vi "Framework Test.vi"() -> ()   [LabVIEW 2017]
uses:
  Builds/Data Sharing Framework/Current/Data Sharing Framework Core/DSF Core.lvlibp/Configuration/Public/Controls/DSF Direction.ctl
  Builds/Data Sharing Framework/Current/Data Sharing Framework Core/DSF Core.lvlibp/Configuration/Public/Controls/DSF Timing Info.ctl
  Builds/Data Sharing Framework/Current/Data Sharing Framework Core/DSF Core.lvlibp/Configuration/Public/Controls/DSF Settings Info.ctl
  Builds/Data Sharing Framework/Current/Data Sharing Framework Core/DSF Core.lvlibp/Configuration/Public/Controls/DSF Data Type.ctl
  <vilib>/Platform/TimedLoop/XDataNode/timing_clust.ctl
  <vilib>/Platform/TimedLoop/XDataNode/nitl_modes.ctl
  <vilib>/Platform/TimedLoop/XDataNode/wakeup.ctl
  Builds/Data Sharing Framework/Current/Data Sharing Framework Core/DSF Core.lvlibp/Engine/Classes/Debug/FIFO Flags/FIFO Flags.lvclass
  Builds/Data Sharing Framework/Current/Data Sharing Framework Core/DSF Core.lvlibp/Engine/Classes/Debug/Debug Flags/Debug Flags.lvclass
  Builds/Data Sharing Framework/Current/Data Sharing Framework Core/DSF Core.lvlibp/Engine/Classes/Framework/Framework.lvclass
  <vilib>/NI/Memory Manager/Classes/Pointer/Pointer.lvclass/Pointer.ctl
  <vilib>/NI/Memory Manager/Classes/Pointer/Public/New/New (4B).vi
  <vilib>/NI/Memory Manager/Classes/Pointer/Public/Write/Write (0D U32).vi
  <vilib>/NI/Memory Manager/Classes/Pointer/Public/New/New (1B).vi
  <vilib>/NI/Memory Manager/Classes/Pointer/Public/Write/Write (0D Bool).vi
  <vilib>/NI/Memory Manager/Classes/Pointer/Public/New/New (8B).vi
  <vilib>/NI/Memory Manager/Classes/Pointer/Public/Read/Read (0D I32).vi
  <vilib>/NI/Memory Manager/Classes/Pointer/Public/Read/Read (0D U32).vi
  <vilib>/NI/Memory Manager/Classes/Pointer/Public/Read/Read (0D Bool).vi
  <vilib>/NI/Memory Manager/Classes/Pointer/Public/Write/Write (0D I32).vi
  <vilib>/NI/Memory Manager/Classes/Pointer/Private/Allocate.vi
  <vilib>/NI/Memory Manager/Classes/Pointer/Public/Write (No Check)/Write (No Check 0D U32).vi
  <vilib>/NI/Memory Manager/Classes/Pointer/Protected/Parameter Checking/Check Null Pointer.vi
  <vilib>/NI/Memory Manager/Classes/Pointer/Protected/Parameter Checking/Check Subset.vi
  <vilib>/NI/Memory Manager/Classes/Pointer/Public/Write (No Check)/Write (No Check 0D Bool).vi
  <vilib>/NI/Memory Manager/Classes/Pointer/Public/Read (No Check)/Read (No Check 0D I32).vi
  <vilib>/NI/Memory Manager/Classes/Pointer/Public/Read (No Check)/Read (No Check 0D U32).vi
  <vilib>/NI/Memory Manager/Classes/Pointer/Public/Read (No Check)/Read (No Check 0D Bool).vi
  <vilib>/NI/Memory Manager/Classes/Pointer/Public/Write (No Check)/Write (No Check 0D I32).vi
  <vilib>/NI/Memory Manager/Classes/Pointer/API/Accessors/Set Address.vi
  <vilib>/NI/Memory Manager/Classes/Pointer/API/Accessors/Set Size.vi
  <vilib>/NI/Memory Manager/Classes/Pointer/Private/Set Internal.vi
  <vilib>/NI/Memory Manager/Classes/Pointer/Protected/Errors.vi
  <vilib>/NI/Memory Manager/Classes/Pointer/Protected/Error VIs/Null Pointer.vi
  <vilib>/NI/Memory Manager/Classes/Pointer/Protected/Error VIs/Out of Bounds.vi
  <vilib>/NI/Memory Manager/Classes/Pointer/Protected/Error Building/Create Error.vi
  <vilib>/NI/Memory Manager/VIs/Write String into Source.vi
  <vilib>/NI/Memory Manager/Classes/Pointer/Protected/Error Building/Write Pointer Size.vi
  <vilib>/NI/Memory Manager/VIs/Write Number into Source.vi
  <vilib>/NI/Memory Manager/VIs/VIs for Poly/Write U64 into Source.vi
  <vilib>/NI/Memory Manager/Constants/Constants.vi
  <vilib>/NI/Memory Manager/Constants/Library Name.vi
  <vilib>/NI/Memory Manager/Classes/Pointer/Protected/Error Building/Get Error Info.vi
  <vilib>/NI/Memory Manager/VIs/Create Error Cluster.vi
  <vilib>/NI/Memory Manager/VIs/VIs for Poly/Create Error Cluster (256B).vi
  <vilib>/NI/Memory Manager/VIs/Set Error Status.vi
  <vilib>/NI/Memory Manager/VIs/Set Error Code.vi
  <vilib>/NI/Memory Manager/VIs/Set Error Source.vi
  <vilib>/NI/Memory Manager/Classes/Pointer/Pointer.lvclass
  <vilib>/platform/TimedLoop/XDataNode/XDataNode.xnode
  <vilib>/Platform/TimedLoop/XDataNode/XDNodeRunTimeDep.lvlib
  Builds/Data Sharing Framework/Current/Data Sharing Framework Core/DSF Core.lvlibp/Engine/Classes/Status/Framework Status.lvclass
  Builds/Data Sharing Framework/Current/Data Sharing Framework Core/DSF Core.lvlibp/Engine/Classes/Status/Framework Performance.lvclass
  Builds/Data Sharing Framework/Current/Data Sharing Framework Core/DSF Core.lvlibp/Configuration/Configuration Session.lvclass
  Builds/Data Sharing Framework/Current/Data Sharing Framework Core/DSF Core.lvlibp
panel:
  in  "Components Path":path=path "C:/Builds/Data Sharing Framework/Windows/32/Transceivers"
  in  "UDP Rx max size":i32=800
  in  "UDP Rx ports":u16[](array[numeric])=[60000, 60001, 60002, 60003]
  in  "Plugins":T5(array[cluster])=[{"plugin class"="UDP", "group configs"=[{"direction"=enum."Tx", "timing"={"priority"=100, "decimation"=1, "offset"=0}, "settings"=[], "transfer configs"=[{"random types?"=FALSE, "non-random type"=enum."DBL", "channel count"=100, "settings"=[{"key"="Destination Address", "value"="localhost"}, {"key"="Destination Port", "value"="60000"}]}]}, {"direction"=enum."Tx", "timing"={"priority"=100, "decimation"=2, "offset"=0}, "settings"=[], "transfer configs"=[{"random types?"=FALSE, "non-random type"=enum."DBL", "channel count"=100, "settings"=[{"key"="Destination Address", "value"="localhost"}, {"key"="Destination Port", "value"="60001"}]}]}, {"direction"=enum."Tx", "timing"={"priority"=100, "decimation"=3, "offset"=0}, "settings"=[], "transfer configs"=[{"random types?"=FALSE, "non-random type"=enum."DBL", "channel count"=100, "settings"=[{"key"="Destination Address", "value"="localhost"}, {"key"="Destination Port", "value"="60002"}]}]}, {"direction"=enum."Tx", "timing"={"priority"=100, "decimation"=4, "offset"=0}, "settings"=[], "transfer configs"=[{"random types?"=FALSE, "non-random type"=enum."DBL", "channel count"=100, "settings"=[{"key"="Destination Address", "value"="localhost"}, {"key"="Destination Port", "value"="60003"}]}]}], "plugin timing"={"priority"=100, "decimation"=1, "offset"=0}, "settings"=[{"key"="Local Port", "value"="50000"}], "thread count"=1}]
  in  "Infinite Timeouts":bool=TRUE
  out "Framework Error":errorcluster
  out "Tx duration":u32 format="%d us"
  out "Rx duration":u32 format="%d us"
  out "Actual Frequency":dbl format="%.0pHz"
  in  "Configuration Path":path=path "C:/github/data-sharing-framework/Testing/test.dsf"
  out "Framework Iteration":i32 format="%d cycles"
  out "Actual Period":u32 format="%d us"
  in  "Target PCL Period":u32=10000 caption="Target Period" format="%d us"
  in  "stop":bool
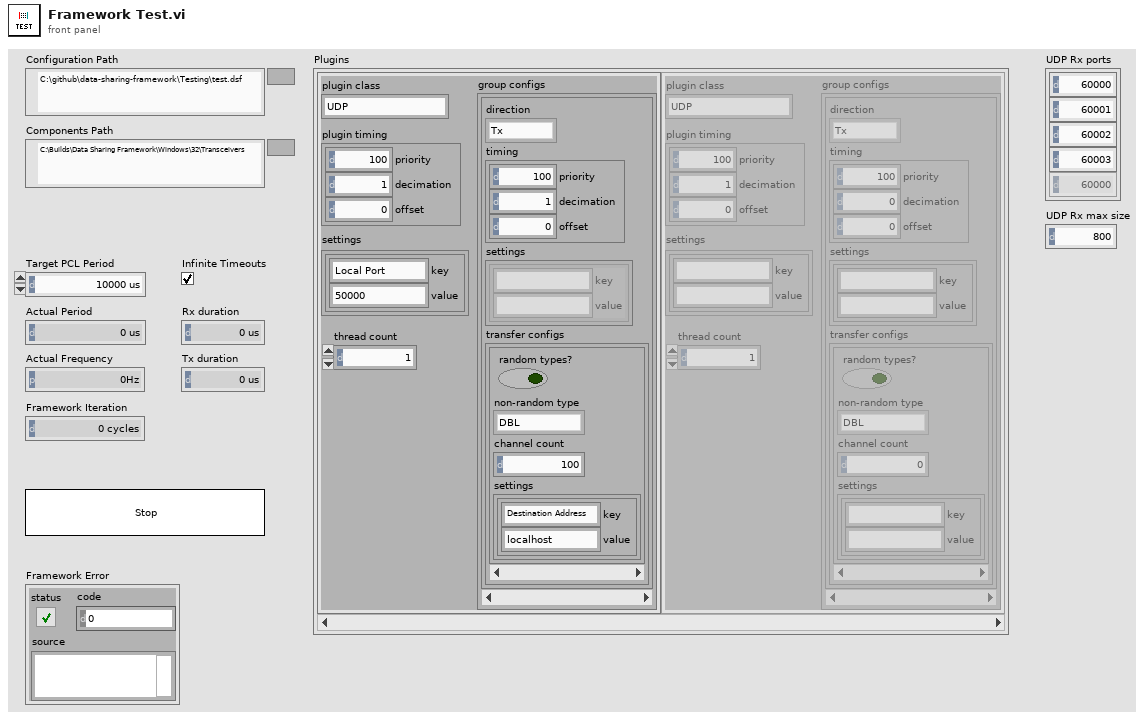
[diagram p1: front panel]
types:
  T1 = typedef "DSF Core.lvlibp/DSF Direction.ctl" = enum8{"Tx", "Rx"}
  T2 = typedef "DSF Core.lvlibp/DSF Timing Info.ctl" = cluster{"priority":u64, "decimation":u64, "offset":u64}
  T3 = typedef "DSF Core.lvlibp/DSF Settings Info.ctl" = cluster{"key":string, "value":string}[]
  T4 = typedef "DSF Core.lvlibp/DSF Data Type.ctl" = enum8{"Bool", "SGL", "DBL", "I8", "I16", "I32", "I64", "U8", "U16", "U32", "U64"}
  T5 = cluster{"plugin class":string, "group configs":cluster{"direction":T1, "timing":T2, "settings":T3, "transfer configs":cluster{"random types?":bool, "non-random type":T4, "channel count":i32, "settings":T3}[]}[], "plugin timing":T2, "settings":T3, "thread count":i32}[]
  T6 = typedef "DSF Core.lvlibp/DSF Engine Framework Configuration.ctl" = cluster{"Plugins":T7[]}
  T7 = typedef "DSF Core.lvlibp/DSF Engine Plugin Configuration.ctl" = cluster{"name":string, "class":string, "cycle timing":T2, "Transfer Groups":T8[], "settings":T3, "thread count":i32}
  T8 = typedef "DSF Core.lvlibp/DSF Engine Transfer Group Configuration.ctl" = cluster{"name":string, "direction":T1, "cycle timing":T2, "Transfers":T9[], "settings":T3}
  T9 = typedef "DSF Core.lvlibp/DSF Engine Transfer Configuration.ctl" = cluster{"name":string, "byte order":T10, "channel configurations":T11[], "settings":T3}
  T10 = typedef "DSF Core.lvlibp/DSF Byte Order.ctl" = enum8{"big-endian", "little-endian"}
  T11 = typedef "DSF Core.lvlibp/DSF Engine Channel Configuration.ctl" = cluster{"engine offset":u64, "name":string, "data type":T4, "count":u64, "buffer offset":u64}
  T12 = typedef "XDNodeRunTimeDep.lvlib/timing_clust.ctl" = cluster{"Expected End [f-1]":u64, "Actual End [f-1]":u64, "Finished Late? [f-1]":bool, "Expected End [i-1]":u64, "Actual End [i-1]":u64, "Finished Late? [i-1]":bool, "Expected Start [i]":u64, "Actual Start [i]":u64, "Expected Start [f]":u64, "Actual Start [f]":u64, "Source Name":string, "Structure Name":string, "Period":i64, "Deadline":i64, "Offset":i64, "Start":i64, "Priority":i32, "Timeout":i32, "Mode":T13, "Wakeup Reason":T14, "Error":errorcluster, "Source Type":string, "Secondary Source Type":string, "Global End Time":u64, "Global Start Time":u64, "Frame Duration":u64, "Iteration Duration":u64, "Assigned CPU":i32, "I/O Scan Engine Mode":u32}
  T13 = typedef "XDNodeRunTimeDep.lvlib/nitl_modes.ctl" = enum32{"No Change", "Process missed periods, maintain original phase", "Discard missed periods, maintain original phase", "Process missed periods, ignore original phase", "Discard missed periods, ignore original phase"}
  T14 = typedef "XDNodeRunTimeDep.lvlib/wakeup.ctl" = enum32{"Normal", "Aborted", "Asynchronous wakeup", "Timing source error", "Timed loop error", "Timeout"}
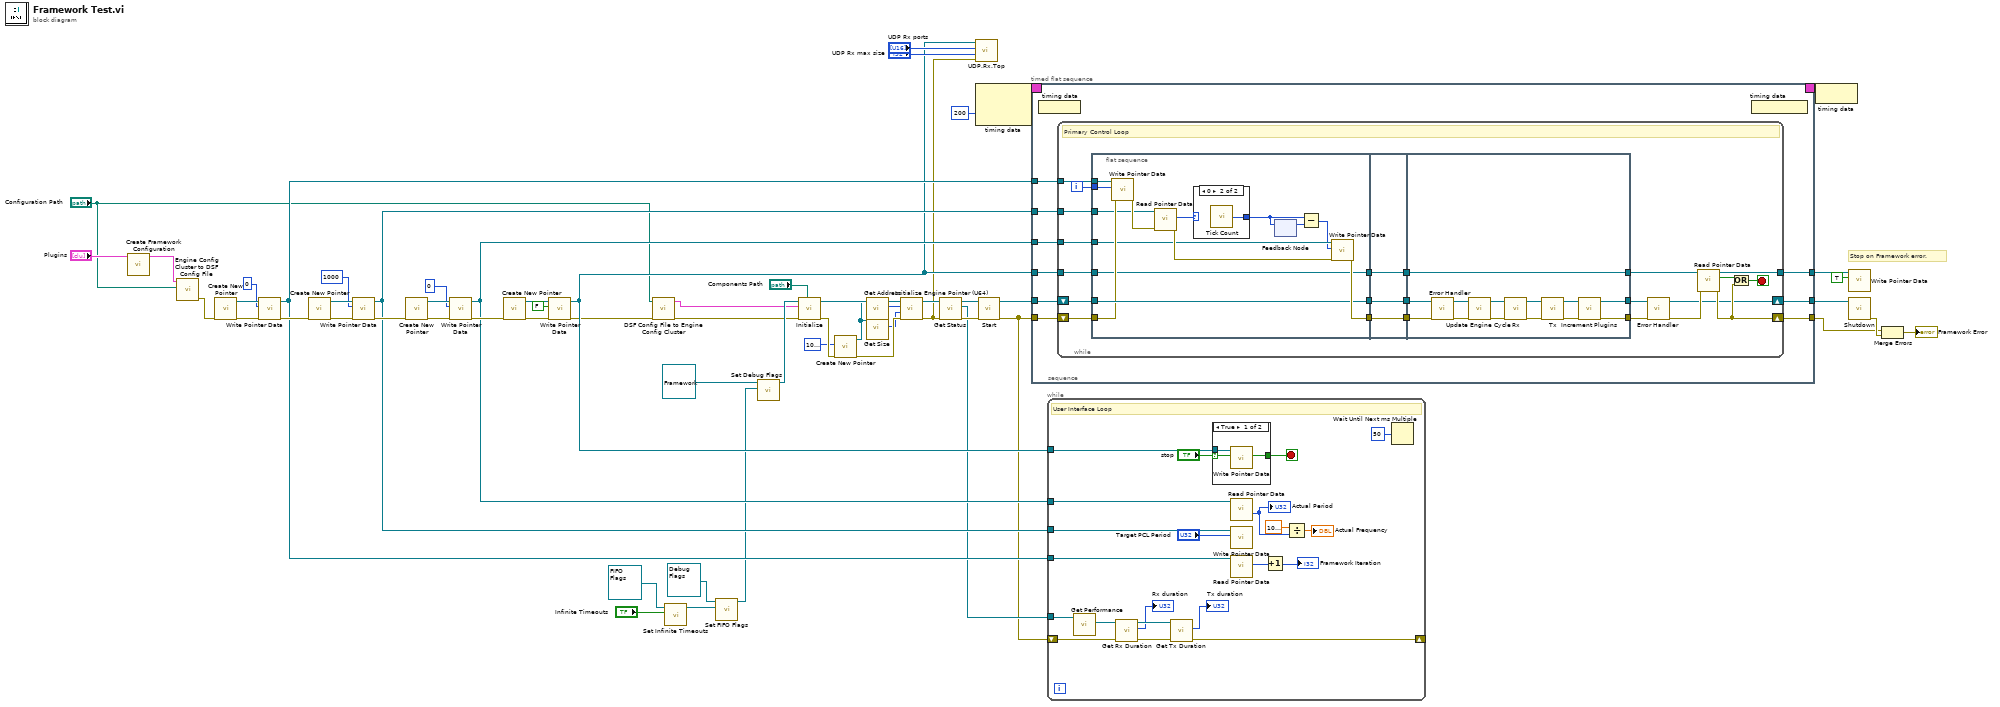
[diagram p0: block diagram]
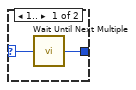
[diagram p2: hidden frame]
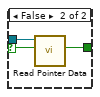
[diagram p3: hidden frame]
diagram:
  # "Stop on Framework error."
  n1 = call "Create Framework Configuration.vi"("Plugins"="Plugins") -> ("Framework Configuration"=w12:T6)  [unwired: 10 in]
  n2 = call "Engine Config Cluster to DSF Config File.vi"("dsf configuration file path"="Configuration Path", "framework configuration"=w12) -> ("error out"=w10:errorcluster)  [unwired: 9 in]
  n3 = call-poly <vilib>:"Create New Pointer.vi"("error in (no error)"=w10) -> ("error out"=w44:errorcluster, "Pointer"=w45:refnum<class "Pointer.lvclass">)  [unwired: 9 in]
  n4 = call-poly <vilib>:"Write Pointer Data.vi"("error in (no error)"=w44, "value"=u32 0, "Pointer in"=w45) -> ("error out"=w43:errorcluster, "Pointer out"=w42:refnum<class "Pointer.lvclass">)  [unwired: 5 in, 2 out]
  n5 = call-poly <vilib>:"Create New Pointer.vi"("error in (no error)"=w43) -> ("error out"=w51:errorcluster, "Pointer"=w52:refnum<class "Pointer.lvclass">)  [unwired: 9 in]
  n6 = call-poly <vilib>:"Write Pointer Data.vi"("error in (no error)"=w51, "value"=u32 1000, "Pointer in"=w52) -> ("error out"=w50:errorcluster, "Pointer out"=w46:refnum<class "Pointer.lvclass">)  [unwired: 5 in, 2 out]
  n7 = call-poly <vilib>:"Create New Pointer.vi"("error in (no error)"=w50) -> ("error out"=w49:errorcluster, "Pointer"=w53:refnum<class "Pointer.lvclass">)  [unwired: 9 in]
  n8 = call-poly <vilib>:"Write Pointer Data.vi"("error in (no error)"=w49, "value"=u32 0, "Pointer in"=w53) -> ("error out"=w48:errorcluster, "Pointer out"=w47:refnum<class "Pointer.lvclass">)  [unwired: 5 in, 2 out]
  n9 = call-poly <vilib>:"Create New Pointer.vi"("error in (no error)"=w48) -> ("error out"=w56:errorcluster, "Pointer"=w55:refnum<class "Pointer.lvclass">)  [unwired: 9 in]
  n10 = call-poly <vilib>:"Write Pointer Data.vi"("error in (no error)"=w56, "value"=FALSE, "Pointer in"=w55) -> ("error out"=w9:errorcluster, "Pointer out"=w37:refnum<class "Pointer.lvclass">)  [unwired: 5 in, 2 out]
  n11 = call "DSF Config File to Engine Config Cluster.vi"("error in (no error)"=w9, "dsf configuration file path"="Configuration Path") -> ("error out"=w8:errorcluster, "framework configuration out"=w13:T6)  [unwired: 8 in]
  n12 = call "Set Infinite Timeouts.vi"("infinite timeouts"="Infinite Timeouts", "FIFO Debug Flags in"=refnum<class "FIFO Flags.lvclass"> refnum ("DSF Core.lvlibp:FIFO Flags.lvclass")) -> ("FIFO Debug Flags out"=w32:refnum<class "FIFO Flags.lvclass">)  [unwired: 9 in]
  n13 = call "Set FIFO Flags.vi"("FIFO"=w32, "Debug Flags in"=refnum<class "Debug Flags.lvclass"> refnum ("DSF Core.lvlibp:Debug Flags.lvclass")) -> ("Debug Flags out"=w30:refnum<class "Debug Flags.lvclass">)  [unwired: 9 in]
  n14 = call "Set Debug Flags.vi"("Debug Flags"=w30, "Framework in"=refnum<class "Framework.lvclass"> refnum ("DSF Core.lvlibp:Framework")) -> ("Framework out"=w29:refnum<class "Framework.lvclass">)  [unwired: 9 in]
  n15 = call "Initialize.vi"("components directory (default)"="Components Path", "error in (no error)"=w8, "framework configuration"=w13, "Framework type"=w29) -> ("error out"=w22:errorcluster, "Framework out"=w25:refnum<class "Framework.lvclass">)  [unwired: 6 in]
  n16 = call-poly <vilib>:"Create New Pointer.vi"("error in (no error)"=w22, "count (1)"=u64 1000000 ("channel count")) -> ("error out"=w21:errorcluster, "Pointer"=w18:refnum<class "Pointer.lvclass">)  [unwired: 8 in]
  n17 = call <vilib>:"Get Address.vi"("Pointer in"=w18) -> ("address"=w20:u64)  [unwired: 9 in, 1 out]
  n18 = call <vilib>:"Get Size.vi"("Pointer in"=w18) -> ("size"=w19:u64)  [unwired: 9 in, 1 out]
  n19 = call "Initialize Engine Pointer (U64).vi"("error in (no error)"=w21, "size"=w19, "address"=w20, "Framework in"=w25) -> ("error out"=w23:errorcluster, "Framework out"=w24:refnum<class "Framework.lvclass">)  [unwired: 6 in]
  n20 = call "Get Status.vi"("Framework in"=w24) -> ("Status"=w14:refnum<class "Framework Status.lvclass">, "Framework out"=w27:refnum<class "Framework.lvclass">)  [unwired: 9 in]
  n21 = call "UDP.Rx.Top.vi"("error in (no error)"=w23, "max size (800)"="UDP Rx max size", "ports"="UDP Rx ports", "Stop Pointer"=w37) -> ()  [unwired: 7 in, 1 out]
  n22 = node-c288(200 ("Priority")) -> (w58:T12)  [unwired: 1 in]
  n23 = call "Start.vi"("error in (no error)"=w23, "Framework in"=w27) -> ("error out"=w7:errorcluster, "Framework out"=w28:refnum<class "Framework.lvclass">)  [unwired: 8 in]
  n24 = timed-sequence {
    timing: w58 -> [_]
    timing-out: [_] -> w57
    tunnel: w28 -> [w67]
    tunnel: w7 -> [w66]
    tunnel: [w65] -> w26
    tunnel: [w64] -> w4
    tunnel: w37 -> [w63]
    tunnel: w46 -> [w62]
    tunnel: w47 -> [w61]
    tunnel: w42 -> [w60]
    tunnel: [w59] -> w36
    n25 = timed-flat-sequence {
      tunnel: w67 -> [w76]
      tunnel: w66 -> [w75]
      tunnel: [w74] -> w65
      tunnel: [w73] -> w64
      tunnel: w63 -> [w72]
      tunnel: w62 -> [w71]
      tunnel: w61 -> [w70]
      tunnel: w60 -> [w69]
      tunnel: [w68] -> w59
      n26 = node-c288() -> ()  [unwired: 1 in]
      n27 = while {
        shift-right: [w77] -> w74
        shift-left: w76 -> [w97]
        shift-right: [w91] -> w73
        shift-left: w75 -> [w98]
        tunnel: w72 -> [w96]
        tunnel: w71 -> [w94]
        tunnel: w70 -> [w93]
        tunnel: w69 -> [w89]
        tunnel: [w81] -> w68
        i -> [w88]
        stop <- w90 stop-if-true
        # "Primary Control Loop"
        n28 = flat-sequence {
          tunnel: w98 -> [w107]
          tunnel: w97 -> [w110]
          tunnel: w96 -> [w103]
          tunnel: [w111] -> w87
          tunnel: [w110] -> w85
          tunnel: [w103] -> w83
          tunnel: w94 -> [w105]
          tunnel: w93 -> [w104]
          tunnel: w89 -> [w108]
          tunnel: w88 -> [w101]
          tunnel: w87 -> [w118]
          tunnel: [w118] -> w86
          tunnel: w85 -> [w117]
          tunnel: [w117] -> w84
          tunnel: w83 -> [w116]
          tunnel: [w116] -> w82
          tunnel: w86 -> [w121]
          tunnel: w84 -> [w122]
          tunnel: w82 -> [w131]
          tunnel: [w131] -> w95
          tunnel: [w124] -> w79
          tunnel: [w123] -> w80
          frame #0 {
            n29 = call-poly <vilib>:"Write Pointer Data.vi"("error in (no error)"=w107, "value"=w101, "Pointer in"=w108) -> ("error out"=w106:errorcluster)  [unwired: 5 in, 3 out]
            n30 = call-poly <vilib>:"Read Pointer Data.vi"("error in (no error)"=w106, "Pointer in"=w105) -> ("error out"=w109:errorcluster, "value out"=w100:u32)  [unwired: 6 in, 2 out]
            n31 = case shown="0" w100 {
              selector: w100 -> [w113 _]
              tunnel: [w114 w115] -> w102
              frame 1.. {
                n32 = call "Wait Until Next Multiple"("Count(uSec)"=w113) -> ("Tick Count(uSec)"=w114:u32)
              }
              frame 0 {
                n33 = call "Tick Count"() -> ("Tick Count(uSec)"=w115:u32)
              }
            }
            n34 = feedback #1() -> (w112:u32)  [unwired: 1 in]
            n35 = feedback-in #1(w102) -> ()
            n36 = Subtract(x=w102, y=w112) -> (x-y=w99:u32)
            n37 = call-poly <vilib>:"Write Pointer Data.vi"("error in (no error)"=w109, "value"=w99, "Pointer in"=w104) -> ("error out"=w111:errorcluster)  [unwired: 5 in, 3 out]
          }
          frame #1 {
          }
          frame #2 {
            n38 = call "Error Handler.vi"("error in (no error)"=w121, "Framework in"=w122) -> ("error out"=w119:errorcluster, "Framework out"=w120:refnum<class "Framework.lvclass">)  [unwired: 8 in]
            n39 = call-dynamic "Update Engine Cycle.vi"("error in (no error)"=w119, "Framework in"=w120) -> ("error out"=w129:errorcluster, "Framework out"=w130:refnum<class "Framework.lvclass">)  [unwired: 8 in]
            n40 = call "Rx.vi"("error in (no error)"=w129, "Framework in"=w130) -> ("error out"=w127:errorcluster, "Framework out"=w128:refnum<class "Framework.lvclass">)  [unwired: 8 in]
            n41 = call "Tx.vi"("error in (no error)"=w127, "Framework in"=w128) -> ("error out"=w126:errorcluster, "Framework out"=w125:refnum<class "Framework.lvclass">)  [unwired: 8 in]
            n42 = call "Increment Plugins.vi"("error in (no error)"=w126, "Framework in"=w125) -> ("error out"=w123:errorcluster, "Framework out"=w124:refnum<class "Framework.lvclass">)  [unwired: 8 in]
          }
        }
        n43 = call "Error Handler.vi"("error in (no error)"=w80, "Framework in"=w79) -> ("error out"=w78:errorcluster, "Framework out"=w77:refnum<class "Framework.lvclass">)  [unwired: 8 in]
        n44 = call-poly <vilib>:"Read Pointer Data.vi"("error in (no error)"=w78, "Pointer in"=w95) -> ("error out"=w91:errorcluster, "value out"=w92:bool, "Pointer out"=w81:refnum<class "Pointer.lvclass">)  [unwired: 6 in, 1 out]
        n45 = Or(x=w92, y=w91) -> (x .or. y?=w90:bool)
      }
      n46 = node-c288() -> ()  [unwired: 1 out]
    }
  }
  n47 = while {
    tunnel: w37 -> [w153]
    tunnel: w47 -> [w150]
    tunnel: w46 -> [w151]
    tunnel: w42 -> [w147]
    tunnel: w14 -> [w143]
    shift-right: [w136] -> _
    shift-left: w7 -> [w138]
    stop <- w154 stop-if-true
    # "User Interface Loop"
    n48 = call "Get Performance.vi"("Framework Status in"=w143) -> ("Framework Performance"=w142:refnum<class "Framework Performance.lvclass">)  [unwired: 9 in, 1 out]
    n49 = call "Get Rx Duration.vi"("error in (no error)"=w138, "Framework Performance in"=w142) -> ("error out"=w137:errorcluster, "rx duration"=→"Rx duration":u32, "Framework Performance out"=w141:refnum<class "Framework Performance.lvclass">)  [unwired: 7 in]
    n50 = call "Get Tx Duration.vi"("error in (no error)"=w137, "Framework Performance in"=w141) -> ("error out"=w136:errorcluster, "tx duration"=→"Tx duration":u32)  [unwired: 7 in, 1 out]
    n51 = case shown="True" "stop" {
      selector: "stop" -> [w155 w158]
      tunnel: [w157 w160] -> w154
      tunnel: w153 -> [w156 w159]
      frame True {
        n52 = call-poly <vilib>:"Write Pointer Data.vi"("value"=w155, "Pointer in"=w156) -> ("value"=w157:bool)  [unwired: 6 in, 3 out]
      }
      frame False {
        n53 = call-poly <vilib>:"Read Pointer Data.vi"("value in"=w158, "Pointer in"=w159) -> ("value out"=w160:bool)  [unwired: 6 in, 3 out]
      }
    }
    n54 = call-poly <vilib>:"Read Pointer Data.vi"("Pointer in"=w150) -> ("offset out"=w145:u64)  [unwired: 7 in, 3 out]
    "Actual Period" <- w145
    n55 = call-poly <vilib>:"Write Pointer Data.vi"("value"="Target PCL Period", "Pointer in"=w151) -> ()  [unwired: 6 in, 4 out]
    n56 = call-poly <vilib>:"Read Pointer Data.vi"("Pointer in"=w147) -> ("value out"=w134:i32)  [unwired: 7 in, 3 out]
    n57 = Increment(x=w134) -> (x+1=→"Framework Iteration":i32)
    n58 = Divide(x=1000000.0, y=w145) -> (x/y=→"Actual Frequency":dbl)
    n59 = Wait Until Next ms Multiple(millisecond multiple=u32 50 ("milliseconds to wait")) -> ()  [unwired: 1 out]
  }
  n60 = node-c288(w57) -> ()
  n61 = call-poly <vilib>:"Write Pointer Data.vi"("value"=TRUE, "Pointer in"=w36) -> ()  [unwired: 6 in, 4 out]
  n62 = call "Shutdown.vi"("Framework in"=w26) -> ("error out"=w6:errorcluster)  [unwired: 9 in, 1 out]
  n63 = Merge Errors(w4, w6) -> (→"Framework Error":errorcluster)
